vi "TestRubikOpGroup.vi"() -> ()   [LabVIEW 2017]
uses:
  <vilib>/myRIO/Common/Instrument Driver Framework/myRIO v1.0/UART/vis/myRIO v1.0 Close UART.vi
  <vilib>/myRIO/Common/Instrument Driver Framework/Utilities/vis/FPGA Ref Manager.vi
  <vilib>/myRIO/Common/Instrument Driver Framework/myRIO v1.0/myRIO v1.0 Reset FPGA.vi
  <vilib>/myRIO/Common/Instrument Driver Framework/myRIO v1.0/IRQ/vis/myRIO v1.0 IRQ Info FGV.vi
  <vilib>/myRIO/Common/Instrument Driver Framework/myRIO v1.0/IRQ/vis/myRIO v1.0 Timer IRQ Info FGV.vi
  <vilib>/myRIO/Common/Instrument Driver Framework/myRIO v1.0/IRQ/vis/myRIO v1.0 ISR Agent.vi
  <vilib>/ErrorRing/Error Ring.xnode
  <vilib>/myRIO/Instrument Drivers/Utilities/Utilities.lvlib
panel:
  out "error out":errorcluster
  # "Executes list of Servo and Grip operations\n\n1) Select device?\n2) If \"Servo\" then angles else not used\n3) If  \"Grip\" then \"closed\"(=T) else not used\n4) Operation is  waiting (synchronous to code)"
  # "Delete one operation: \nRightmouse click@element > Data Operations > Delete element\n\nIf item is not enabled then operation is not executed\n\nSave operations:\nRightmouse click@array > Data Operations > Make current value default\n\nReinitialize:\nRightmouse click@array > Data Operations > Reinitialize"
  # "At Start list of operations will pop up!"
  # "1sec delay in for-loop!"
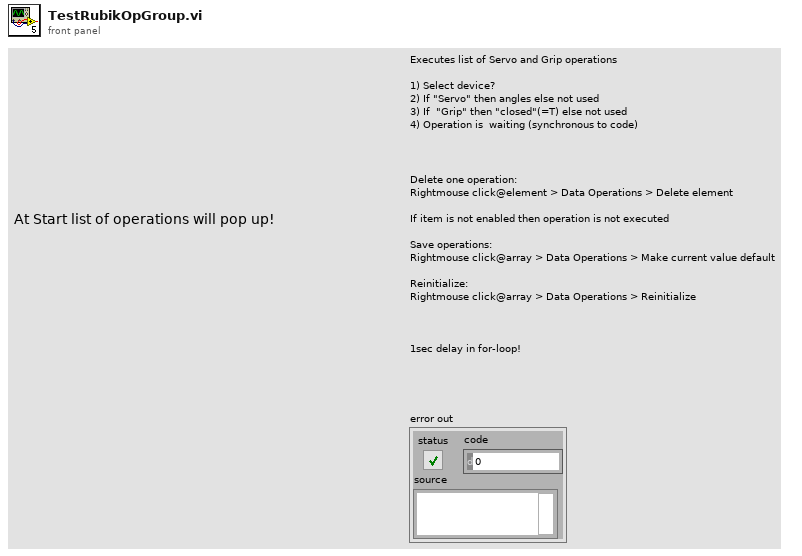
[diagram p1: front panel]
types:
  T1 = typedef "RubikLibrary.lvlib/RubikOps.ctl" = cluster{"Device":enum16{"Servo", "SyncTurn", "Grip"}, "Angles":T2[], "Grips":bool[], "NoWaits":bool[]}
  T2 = typedef "RubikLibrary.lvlib/ServoAbsAngleControl.ctl" = enum16{"+90°", "0°", "-90°"}
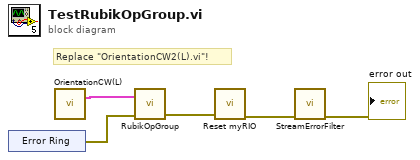
[diagram p0: block diagram]
diagram:
  # "Replace \"OrientationCW2(L).vi\"!"
  n1 = xnode "Error Ring"() -> ("error out"=w5:errorcluster)
  n2 = call "OrientationCW(L).vi"() -> ("Array of Operations (out)"=w1:T1[])  [unwired: 2 in]
  n3 = call "RubikOpGroup.vi"("error in"=w5, "Array of Operations"=w1) -> ("error out"=w3:errorcluster)  [unwired: 1 in]
  n4 = call <vilib>:"Reset myRIO.vi"("error in (no error)"=w3) -> ("error out"=w2:errorcluster)  [unwired: 10 in]
  n5 = call "StreamErrorFilter.vi"("error in (no error)"=w2) -> ("error out"=→"error out":errorcluster)  [unwired: 10 in]
